vi "update-image-data-on-trace.vi"(9 "iterator":i32, 10 "master-image-data-n":dbl[][](array[numeric]), 11 "avg-data-row":dbl[](array[numeric])) -> (3 "master-image-data-out":dbl[][](array[numeric]))   [LabVIEW 2015]
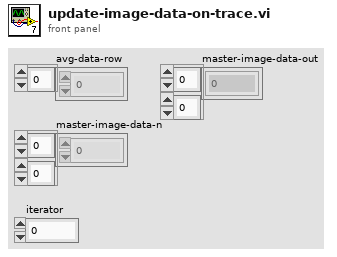
[diagram p1: front panel]
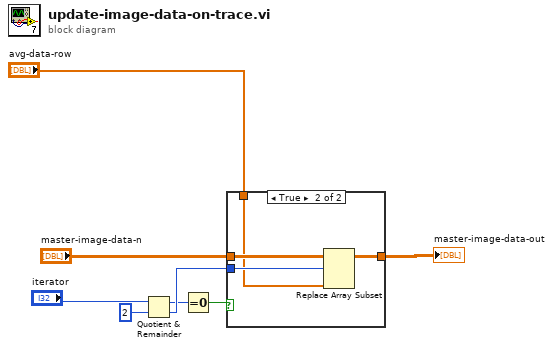
[diagram p0: block diagram]
diagram:
  n1 = Quotient & Remainder(x="iterator", y=2) -> (x-y*floor(x/y)=w7:i32, floor(x/y)=w8:i32)
  n2 = Equal To 0?(x=w7) -> (x = 0?=w6:bool)
  n3 = case shown="True" w6 {
    tunnel: w8 -> [_ w13]
    tunnel: [w9 w12] -> w1
    tunnel: "master-image-data-n" -> [w9 w11]
    tunnel: "avg-data-row" -> [_ w10]
    frame False {
    }
    frame True {
      n4 = Replace Array Subset(array=w11, new element=w10, index (row)=w13) -> (w12:dbl[][])  [unwired: 1 in]
    }
  }
  "master-image-data-out" <- w1
